vi "Manual_range_select.vi"(9 "CH1":u8(knob) scale=0.0..3.0, 10 "EN":bool, 11 "CH0":u8(knob) scale=0.0..3.0) -> (2 "CH0 control 2":string, 3 "CH0 control":string)   [LabVIEW 2012]
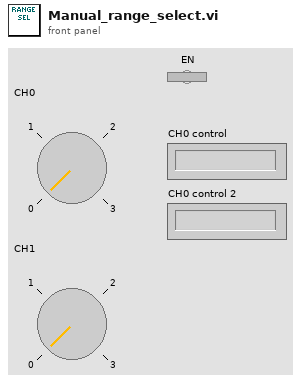
[diagram p1: front panel]
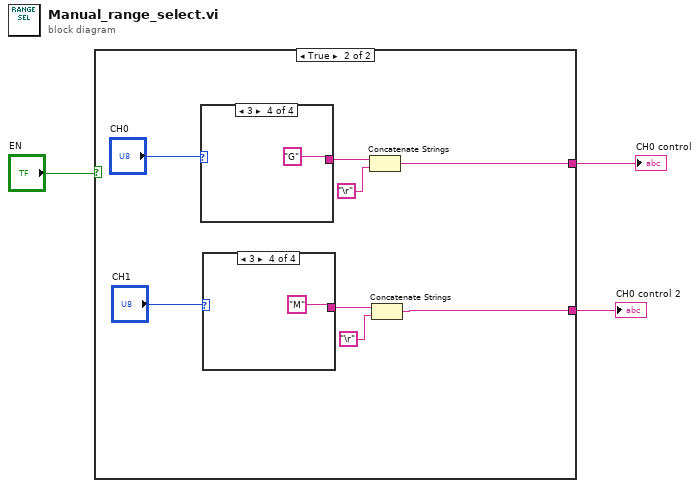
[diagram p0: block diagram]
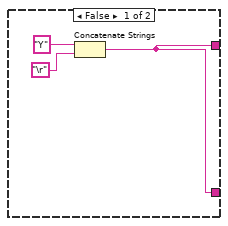
[diagram p2: hidden frame]
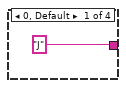
[diagram p3: hidden frame]
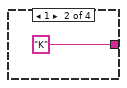
[diagram p4: hidden frame]
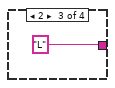
[diagram p5: hidden frame]
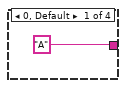
[diagram p6: hidden frame]
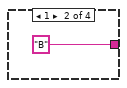
[diagram p7: hidden frame]
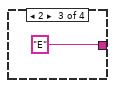
[diagram p8: hidden frame]
diagram:
  n1 = case shown="True" "EN" {
    tunnel: [w4 w11] -> w2
    tunnel: [w4 w7] -> w1
    frame False {
      n2 = Concatenate Strings("Y", "\r") -> (w4:string)
    }
    frame True {
      n3 = case shown="3" "CH0" {
        tunnel: ["A" "B" "E" "G"] -> w13
        frame 0, Default {
        }
        frame 1 {
        }
        frame 2 {
        }
        frame 3 {
        }
      }
      n4 = case shown="3" "CH1" {
        tunnel: ["J" "K" "L" "M"] -> w9
        frame 0, Default {
        }
        frame 1 {
        }
        frame 2 {
        }
        frame 3 {
        }
      }
      n5 = Concatenate Strings(w13, "\r") -> (w11:string)
      n6 = Concatenate Strings(w9, "\r") -> (w7:string)
    }
  }
  "CH0 control" <- w2
  "CH0 control 2" <- w1
